vi "Add_to_store.vi"(6 "Store":T1=enum."command", 8 "error in (no error)":errorcluster, 10 "Waveform":waveform(dbl), 11 "RFID system in":refnum<class "RFID system.lvclass">) -> (0 "error out":errorcluster, 3 "RFID system out":refnum<class "RFID system.lvclass">)   [LabVIEW 2019, in "RFID system.lvclass"]
uses:
  RFID system.lvclass
  TypeDef/Store.ctl
  Support VI's/Write waveform.vi
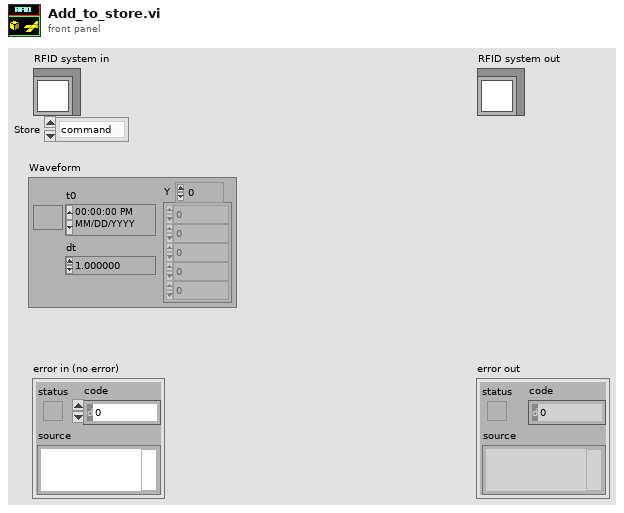
[diagram p1: front panel]
types:
  T1 = typedef "Store.ctl" = enum16{"envelope", "noise", "demSubCar", "CH_frame", "Decode", "demodulate", "in", "out", "sum", "subCarrier", "frame", "command", "encode", "modulate", "encode_UP", "modulate_up", "demod_up", "envelop_up", "sum_up", "out_up", "in_up"}
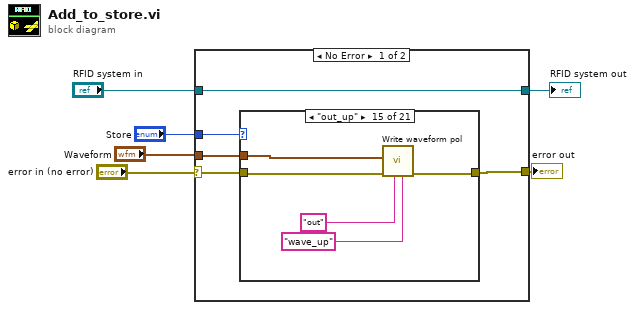
[diagram p0: block diagram]
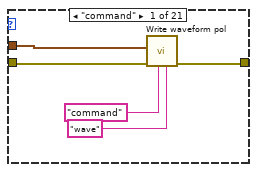
[diagram p2: hidden frame]
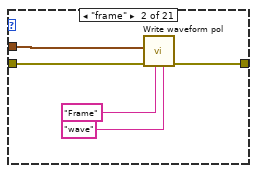
[diagram p3: hidden frame]
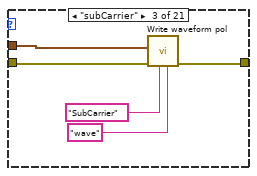
[diagram p4: hidden frame]
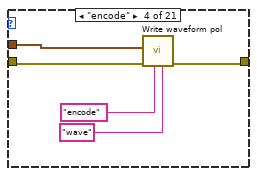
[diagram p5: hidden frame]
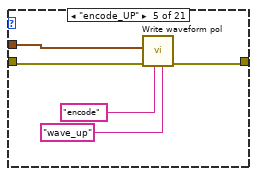
[diagram p6: hidden frame]
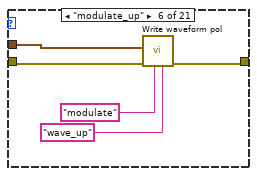
[diagram p7: hidden frame]
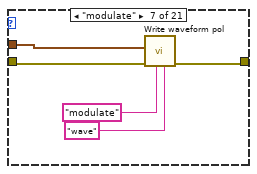
[diagram p8: hidden frame]
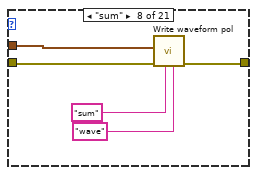
[diagram p9: hidden frame]
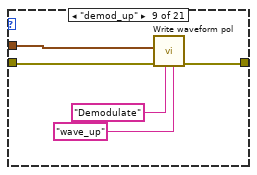
[diagram p10: hidden frame]
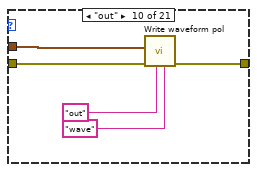
[diagram p11: hidden frame]
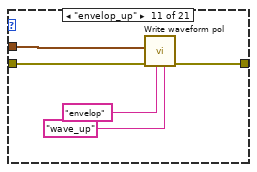
[diagram p12: hidden frame]
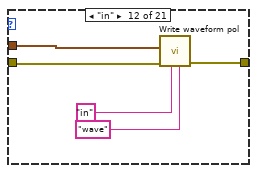
[diagram p13: hidden frame]
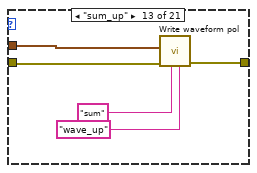
[diagram p14: hidden frame]
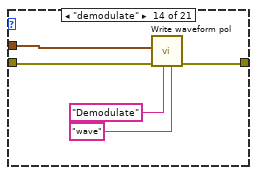
[diagram p15: hidden frame]
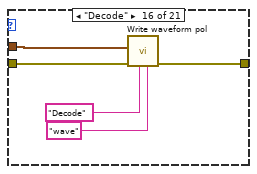
[diagram p16: hidden frame]
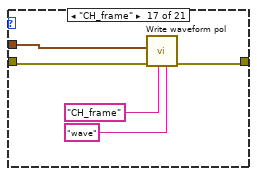
[diagram p17: hidden frame]
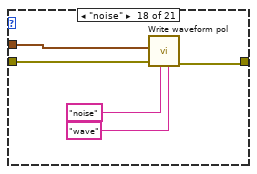
[diagram p18: hidden frame]
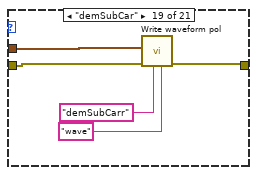
[diagram p19: hidden frame]
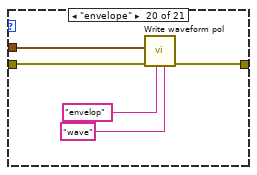
[diagram p20: hidden frame]
diagram:
  n1 = case shown="No Error" "error in (no error)" {
    selector: "error in (no error)" -> [w8 w118]
    tunnel: [w7 w118] -> w5
    tunnel: [w11 w117] -> w3
    tunnel: "RFID system in" -> [w11 w117]
    tunnel: "Waveform" -> [w10 _]
    tunnel: "Store" -> [w9 _]
    frame No Error {
      n2 = case shown="\"out_up\"" w9 {
        tunnel: w10 -> [w14 w19 w24 w29 w34 w39 w44 w49 w54 w59 w64 w69 w74 w79 w84 w91 w94 w99 w104 w109 w114]
        tunnel: w8 -> [w15 w20 w25 w30 w35 w40 w45 w50 w55 w60 w65 w70 w75 w80 w85 w90 w95 w100 w105 w110 w115]
        tunnel: [w13 w18 w23 w28 w33 w38 w43 w48 w53 w58 w63 w68 w73 w78 w83 w89 w93 w98 w103 w108 w113] -> w7
        frame "command" {
          n3 = call-poly "Write waveform pol.vi"("Channel"="wave", "Name note"="command", "error in (no error)"=w15, "Waveform"=w14) -> ("error out"=w13:errorcluster)  [unwired: 7 in]
        }
        frame "frame" {
          n4 = call-poly "Write waveform pol.vi"("Channel"="wave", "Name note"="Frame", "error in (no error)"=w20, "Waveform"=w19) -> ("error out"=w18:errorcluster)  [unwired: 7 in]
        }
        frame "subCarrier" {
          n5 = call-poly "Write waveform pol.vi"("Channel"="wave", "Name note"="SubCarrier", "error in (no error)"=w25, "Waveform"=w24) -> ("error out"=w23:errorcluster)  [unwired: 7 in]
        }
        frame "encode" {
          n6 = call-poly "Write waveform pol.vi"("Channel"="wave", "Name note"="encode", "error in (no error)"=w30, "Waveform"=w29) -> ("error out"=w28:errorcluster)  [unwired: 7 in]
        }
        frame "encode_UP" {
          n7 = call-poly "Write waveform pol.vi"("Channel"="wave_up", "Name note"="encode", "error in (no error)"=w35, "Waveform"=w34) -> ("error out"=w33:errorcluster)  [unwired: 7 in]
        }
        frame "modulate_up" {
          n8 = call-poly "Write waveform pol.vi"("Channel"="wave_up", "Name note"="modulate", "error in (no error)"=w40, "Waveform"=w39) -> ("error out"=w38:errorcluster)  [unwired: 7 in]
        }
        frame "modulate" {
          n9 = call-poly "Write waveform pol.vi"("Channel"="wave", "Name note"="modulate", "error in (no error)"=w45, "Waveform"=w44) -> ("error out"=w43:errorcluster)  [unwired: 7 in]
        }
        frame "sum" {
          n10 = call-poly "Write waveform pol.vi"("Channel"="wave", "Name note"="sum", "error in (no error)"=w50, "Waveform"=w49) -> ("error out"=w48:errorcluster)  [unwired: 7 in]
        }
        frame "demod_up" {
          n11 = call-poly "Write waveform pol.vi"("Channel"="wave_up", "Name note"="Demodulate", "error in (no error)"=w55, "Waveform"=w54) -> ("error out"=w53:errorcluster)  [unwired: 7 in]
        }
        frame "out" {
          n12 = call-poly "Write waveform pol.vi"("Channel"="wave", "Name note"="out", "error in (no error)"=w60, "Waveform"=w59) -> ("error out"=w58:errorcluster)  [unwired: 7 in]
        }
        frame "envelop_up" {
          n13 = call-poly "Write waveform pol.vi"("Channel"="wave_up", "Name note"="envelop", "error in (no error)"=w65, "Waveform"=w64) -> ("error out"=w63:errorcluster)  [unwired: 7 in]
        }
        frame "in" {
          n14 = call-poly "Write waveform pol.vi"("Channel"="wave", "Name note"="in", "error in (no error)"=w70, "Waveform"=w69) -> ("error out"=w68:errorcluster)  [unwired: 7 in]
        }
        frame "sum_up" {
          n15 = call-poly "Write waveform pol.vi"("Channel"="wave_up", "Name note"="sum", "error in (no error)"=w75, "Waveform"=w74) -> ("error out"=w73:errorcluster)  [unwired: 7 in]
        }
        frame "demodulate" {
          n16 = call-poly "Write waveform pol.vi"("Channel"="wave", "Name note"="Demodulate", "error in (no error)"=w80, "Waveform"=w79) -> ("error out"=w78:errorcluster)  [unwired: 7 in]
        }
        frame "out_up" {
          n17 = call-poly "Write waveform pol.vi"("Channel"="wave_up", "Name note"="out", "error in (no error)"=w85, "Waveform"=w84) -> ("error out"=w83:errorcluster)  [unwired: 7 in]
        }
        frame "Decode" {
          n18 = call-poly "Write waveform pol.vi"("Channel"="wave", "Name note"="Decode", "error in (no error)"=w90, "Waveform"=w91) -> ("error out"=w89:errorcluster)  [unwired: 7 in]
        }
        frame "CH_frame" {
          n19 = call-poly "Write waveform pol.vi"("Channel"="wave", "Name note"="CH_frame", "error in (no error)"=w95, "Waveform"=w94) -> ("error out"=w93:errorcluster)  [unwired: 7 in]
        }
        frame "noise" {
          n20 = call-poly "Write waveform pol.vi"("Channel"="wave", "Name note"="noise", "error in (no error)"=w100, "Waveform"=w99) -> ("error out"=w98:errorcluster)  [unwired: 7 in]
        }
        frame "demSubCar" {
          n21 = call-poly "Write waveform pol.vi"("Channel"="wave", "Name note"="demSubCarr", "error in (no error)"=w105, "Waveform"=w104) -> ("error out"=w103:errorcluster)  [unwired: 7 in]
        }
        frame "envelope" {
          n22 = call-poly "Write waveform pol.vi"("Channel"="wave", "Name note"="envelop", "error in (no error)"=w110, "Waveform"=w109) -> ("error out"=w108:errorcluster)  [unwired: 7 in]
        }
        frame "in_up" {
          n23 = call-poly "Write waveform pol.vi"("Channel"="wave_up", "Name note"="in", "error in (no error)"=w115, "Waveform"=w114) -> ("error out"=w113:errorcluster)  [unwired: 7 in]
        }
      }
    }
    frame Error {
    }
  }
  "error out" <- w5
  "RFID system out" <- w3
